vi "Byte69_82 (SubVI).vi"(1 "Card Number":dbl, 2 "Input String":string) -> (0 "Cluster":T1)   [LabVIEW 2024]
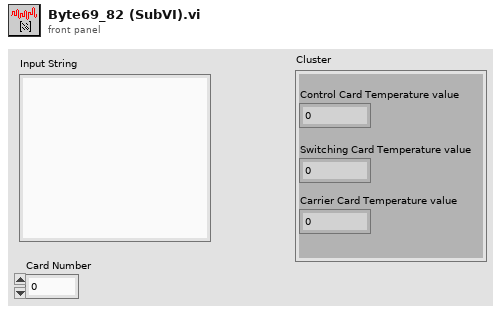
[diagram p1: front panel]
types:
  T1 = cluster{"Control Card Temperature value ":dbl, "Switching Card Temperature value":dbl, "Carrier Card Temperature value":dbl}
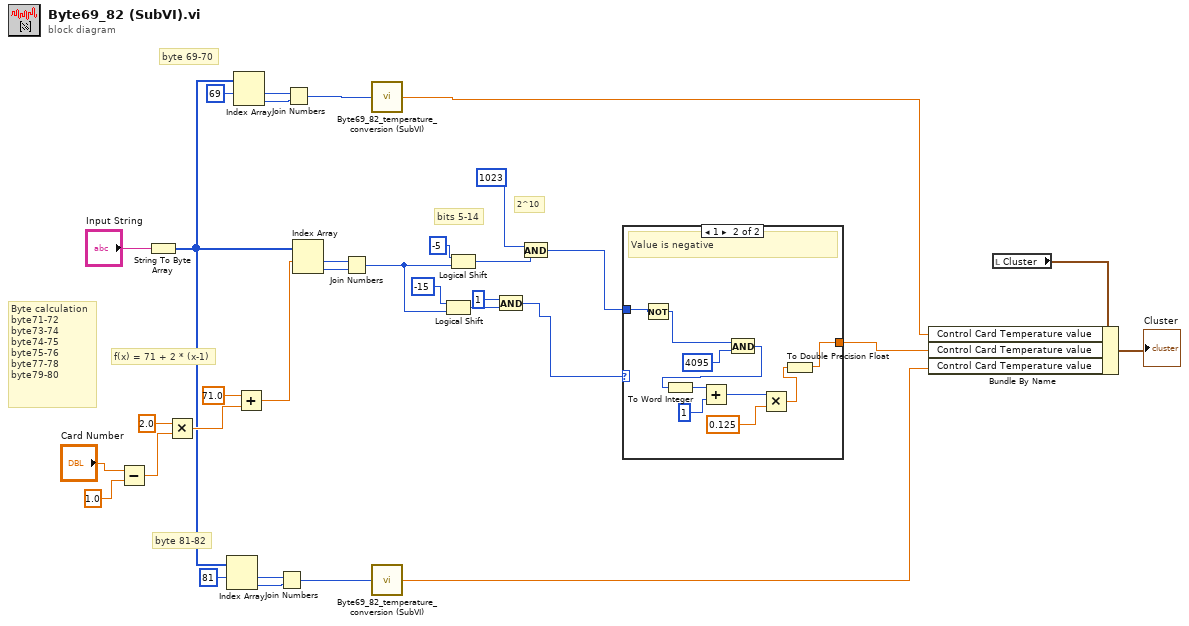
[diagram p0: block diagram]
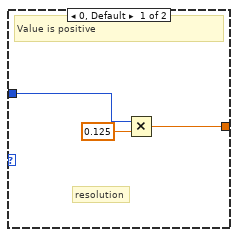
[diagram p2: hidden frame]
diagram:
  # "byte 81-82"
  # "Byte calculation\nbyte71-72\nbyte73-74\nbyte74-75\nbyte75-76\nbyte77-78\nbyte79-80"
  # "f(x) = 71 + 2 * (x-1)"
  # "2^10"
  # "bits 5-14"
  # "byte 69-70"
  n1 = Subtract(x="Card Number", y=1.0) -> (x-y=w14:dbl)
  n2 = String To Byte Array(string="Input String") -> (unsigned byte array=w8:u8[])
  n3 = Multiply(x=2.0, y=w14) -> (x*y=w13:dbl)
  n4 = Index Array "Index Array"(array=w8, index #1=81 ("index")) -> (element #1=w9:u8, element #2=w10:u8)  [unwired: 1 in]
  n5 = Index Array "Index Array"(array=w8, index #1=69 ("index")) -> (element #1=w31:u8, element #2=w32:u8)  [unwired: 1 in]
  n6 = Add(x=71.0, y=w13) -> (x+y=w12:dbl)
  n7 = Join Numbers(hi=w9, lo=w10) -> ((hi.lo)=w6:u16)
  n8 = Join Numbers(hi=w31, lo=w32) -> ((hi.lo)=w30:u16)
  n9 = Index Array "Index Array"(array=w8, index #1=w12) -> (element #1=w26:u8, element #2=w27:u8)  [unwired: 1 in]
  n10 = Join Numbers(hi=w26, lo=w27) -> ((hi.lo)=w18:u16)
  n11 = call "Byte69_82_temperature_conversion (SubVI).vi"("Numeric"=w30) -> ("Control Card Temperature value"=w3:dbl)
  n12 = call "Byte69_82_temperature_conversion (SubVI).vi"("Numeric"=w6) -> ("Control Card Temperature value"=w1:dbl)
  n13 = Logical Shift(y=i16 -15, x=w18) -> (x << y=w22:u16)
  n14 = Logical Shift(y=i16 -5, x=w18) -> (x << y=w25:u16)
  n15 = And(x=u16 1, y=w22) -> (x .and. y?=w20:u16)
  n16 = And(x=u16 1023, y=w25) -> (x .and. y?=w19:u16)
  n17 = case shown="1" w20 {
    tunnel: w19 -> [w36 w38]
    tunnel: [w34 w37] -> w2
    frame 0, Default {
      # "resolution"
      # "Value is positive"
      n18 = Multiply(x=w36, y=0.125) -> (x*y=w34:dbl)
    }
    frame 1 {
      # "Value is negative"
      n19 = Not(x=w38) -> (.not. x?=w42:u16)
      n20 = And(x=w42, y=u16 4095) -> (x .and. y?=w40:u16)
      n21 = To Word Integer(number=w40) -> (16bit integer=w39:i16)
      n22 = Add(x=w39, y=i16 1) -> (x+y=w45:i16)
      n23 = Multiply(x=w45, y=0.125) -> (x*y=w43:dbl)
      n24 = To Double Precision Float(number=w43) -> (double precision float=w37:dbl)
    }
  }
  n25 = local read "Cluster"() -> (w5:T1)
  n26 = Bundle By Name(cluster=w5, "Control Card Temperature value"=w3, "Control Card Temperature value"=w2, "Control Card Temperature value"=w1) -> (→"Cluster":T1)
